vi "HEWH Check AO Values.vi"(8 "error in (no error)":errorcluster, 10 "Module 4 Relay Status Input":T1, 11 "VISA session":refnum<visa-resource-name>="MW100") -> (0 "error out":errorcluster, 2 "Module 4 Relay Status Output":T1, 3 "dup VISA session":refnum<visa-resource-name>)   [LabVIEW 2023]
uses:
  Type Definitions/HEWH Module 4 Relay Status.ctl
  Type Definitions/HEWH MW100 Channel Numbers.ctl
panel:
  out "Data Status List":T2(array[ring])
  out "Unit List":string[](array[string])
  out "Data List (Debug)":dbl[](array[numeric])
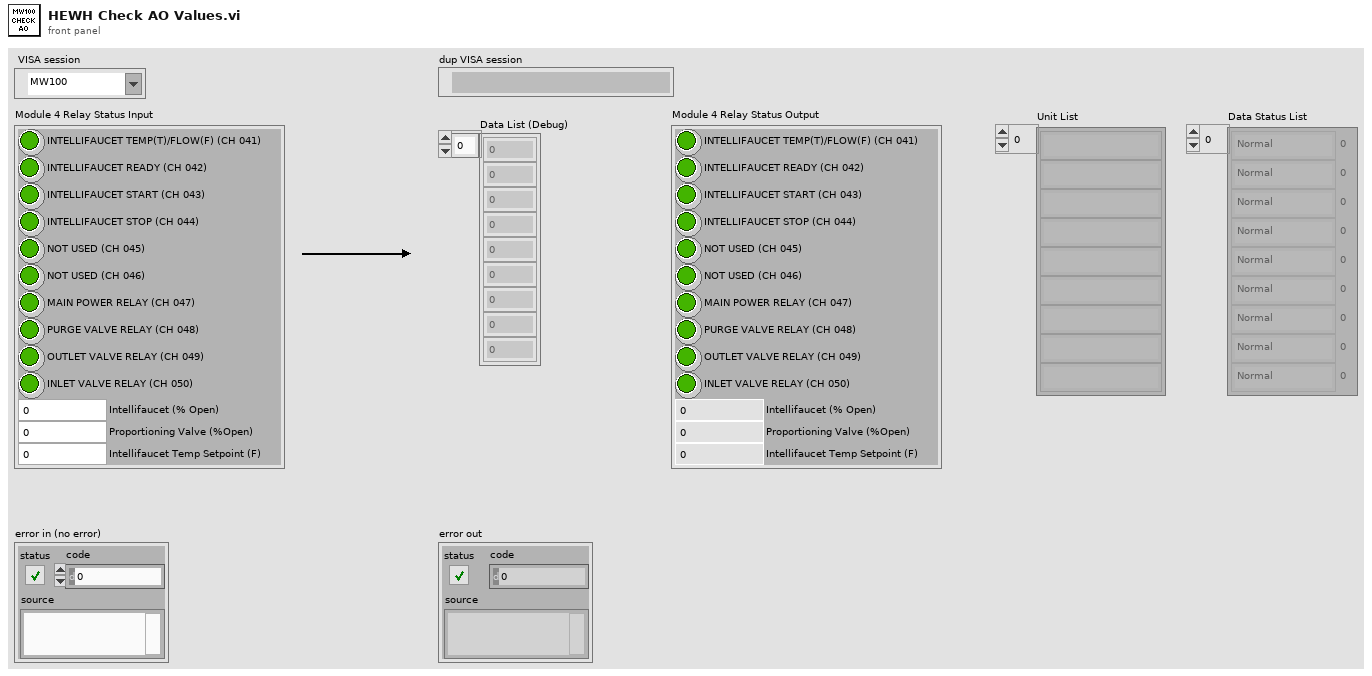
[diagram p1: front panel]
types:
  T1 = typedef "HEWH Module 4 Relay Status.ctl" = cluster{"INTELLIFAUCET TEMP(T)/FLOW(F) (CH 041)":bool, "INTELLIFAUCET READY (CH 042)":bool, "INTELLIFAUCET START (CH 043)":bool, "INTELLIFAUCET STOP (CH 044)":bool, "MAIN POWER RELAY (CH 047)":bool, "NOT USED (CH 045)":bool, "NOT USED (CH 046)":bool, "PURGE VALVE RELAY (CH 048)":bool, "OUTLET VALVE RELAY (CH 049)":bool, "INLET VALVE RELAY (CH 050)":bool, "Intellifaucet (% Open)":dbl, "Proportioning Valve (%Open)":dbl, "Intellifaucet Temp Setpoint (F)":dbl}
  T2 = enum8{"Normal", "Differential Input", "Skip", "Over", "Error"}[]
  T3 = typedef "HEWH MW100 Channel Numbers.ctl" = string
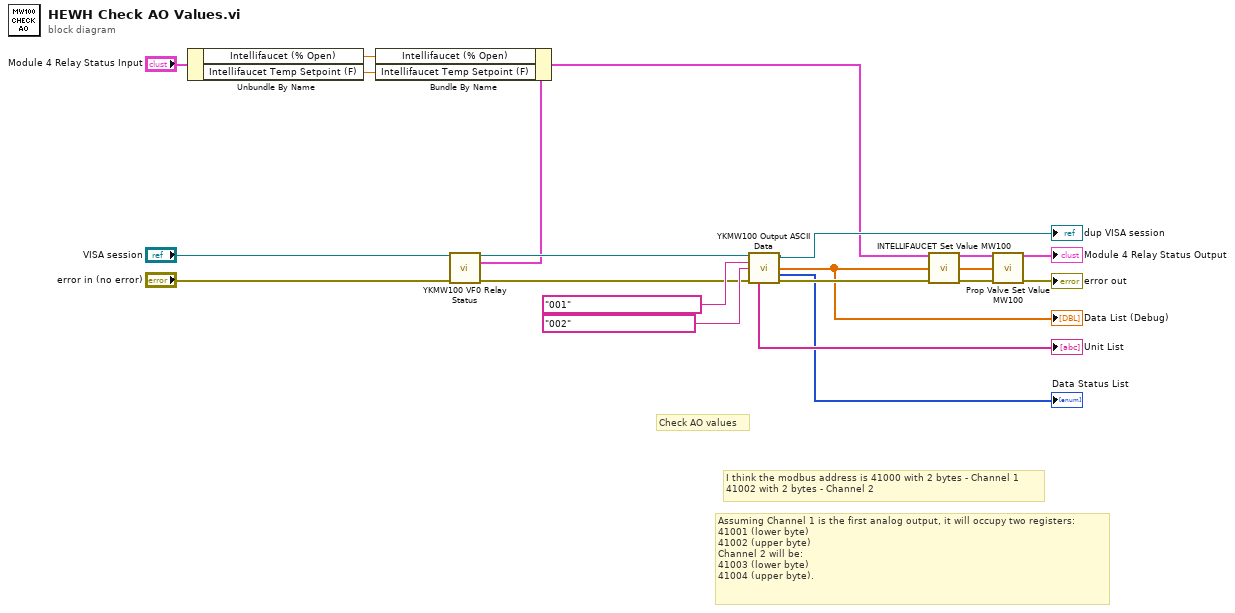
[diagram p0: block diagram]
diagram:
  # "Assuming Channel 1 is the first analog output, it will occupy two registers:\n41001 (lower byte)\n41002 (upper byte)\nChannel 2 will be:\n41003 (lower byte)\n41004 (upper byte)."
  # "I think the modbus address is 41000 with 2 bytes - Channel 1\n41002 with 2 bytes - Channel 2"
  # "Check AO values"
  n1 = Unbundle By Name("Module 4 Relay Status Input") -> ("Intellifaucet (% Open)"=w2:dbl, "Intellifaucet Temp Setpoint (F)"=w1:dbl)
  n2 = call "YKMW100 VF0 Relay Status.vi"("MW100"="VISA session", "Error In"="error in (no error)") -> ("MW100 Out"=w9:refnum<visa-resource-name>, "Module 4 Relay Status"=w4:T1, "error out"=w10:errorcluster)  [unwired: 9 in, 2 out]
  n3 = Bundle By Name(cluster=w4, "Intellifaucet (% Open)"=w2, "Intellifaucet Temp Setpoint (F)"=w1) -> (w3:T1)
  n4 = call "YKMW100 Output ASCII Data.vi"("VISA session"=w9, "Start Channel (001)"=T3 "001" ("Output Start"), "End Channel (001)"=T3 "002" ("Output End"), "error in (no error)"=w10) -> ("dup VISA session"=→"dup VISA session":refnum<visa-resource-name>, "Data List"=w12:dbl[], "Data Status List"=→"Data Status List":T2, "Unit List"=→"Unit List":string[], "error out"=w17:errorcluster)  [unwired: 5 in, 2 out]
  "Data List (Debug)" <- w12
  n5 = call "INTELLIFAUCET Set Value MW100.vi"("Module 4 Relay Status Input"=w3, "AO Data"=w12, "error in (no error)"=w17) -> ("Module 4 Relay Status Output"=w14:T1, "AO Data Output"=w11:dbl[], "error out"=w16:errorcluster)  [unwired: 10 in]
  n6 = call "Prop Valve Set Value MW100.vi"("Module 4 Relay Status Input"=w14, "AO Data"=w11, "error in (no error)"=w16) -> ("Module 4 Relay Status Output"=→"Module 4 Relay Status Output":T1, "error out"=→"error out":errorcluster)  [unwired: 11 in]
